vi "Start Cooker.vi"(8 "error in (no error)":errorcluster, 11 "Kitchen Actor in":refnum<class "Kitchen Actor.lvclass">) -> (0 "error out":errorcluster, 3 "Kitchen Actor out":refnum<class "Kitchen Actor.lvclass">)   [LabVIEW 2024, in "Kitchen Actor.lvlib" / "Kitchen Actor.lvclass"]
uses:
  Kitchen Actor.lvclass
  Kitchen Actor.lvclass/Kitchen Actor.ctl
  <vilib>/numeric/Random Number (Range) DBL.vi
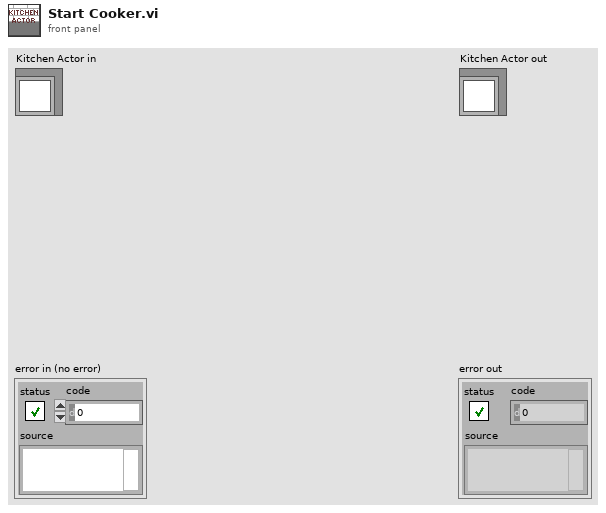
[diagram p1: front panel]
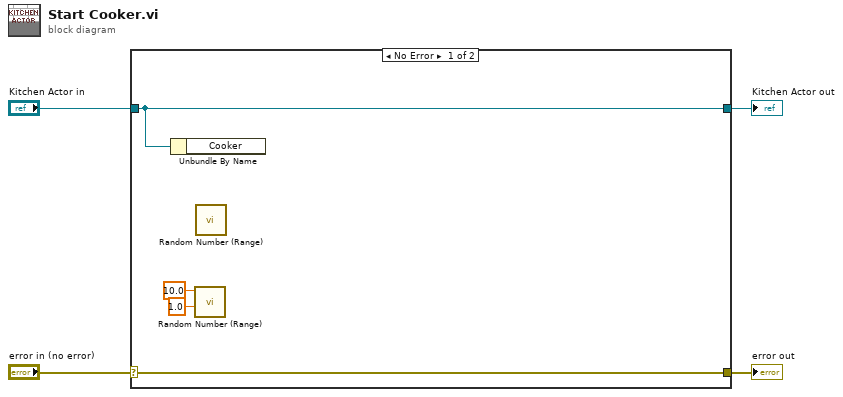
[diagram p0: block diagram]
diagram:
  n1 = case shown="No Error" "error in (no error)" {
    selector: "error in (no error)" -> [w5 w10]
    tunnel: [w5 w10] -> w3
    tunnel: [w8 w9] -> w1
    tunnel: "Kitchen Actor in" -> [w8 w9]
    frame No Error {
      n2 = Unbundle By Name(w8) -> ()  [unwired: 1 out]
      n3 = call-poly <vilib>:"Random Number (Range).vi"("lower bound (0)"=1.0, "upper bound (100)"=10.0) -> ()  [unwired: 9 in, 1 out]
      n4 = call-poly <vilib>:"Random Number (Range).vi"() -> ()  [unwired: 11 in, 1 out]
    }
    frame Error {
    }
  }
  "error out" <- w3
  "Kitchen Actor out" <- w1
